vi "Error - Log File.vi"(6 "Clear error?":bool, 8 "error in":errorcluster) -> (0 "error out":errorcluster)   [LabVIEW 2017]
doc: "This SubVI create new or add to existing text file (error_log.txt) data about occured error and current timestamp. Also user can clear occured error by boolean control \"Clear?\"."
uses:
  <vilib>/ErrorRing/Error Ring.xnode
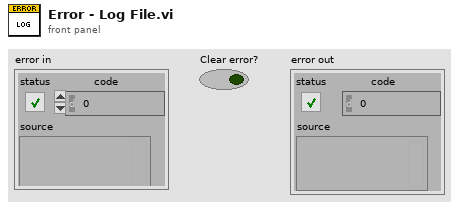
[diagram p1: front panel]
types:
  T1 = enum16{"open", "replace", "create", "open or create", "replace or create", "replace or create with confirmation"}
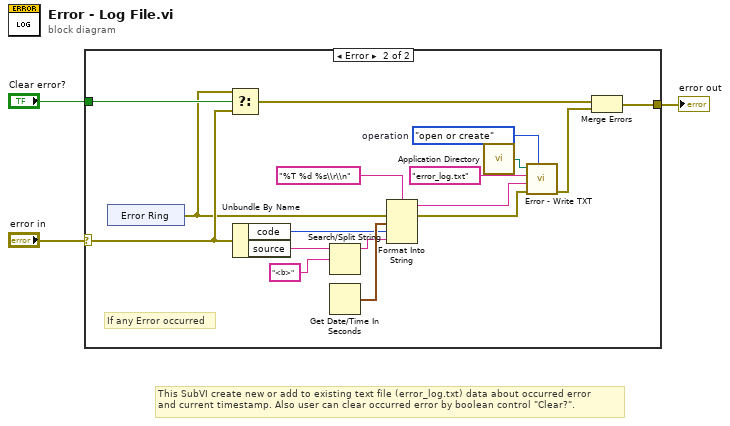
[diagram p0: block diagram]
diagram:
  # "This SubVI create new or add to existing text file (error_log.txt) data about occurred error \nand current timestamp. Also user can clear occurred error by boolean control \"Clear?\"."
  n1 = case shown="Error" "error in" {
    selector: "error in" -> [w4 w13]
    tunnel: [w4 w14] -> w3
    tunnel: "Clear error?" -> [_ w12]
    frame No Error {
      # "If NO Error occurred"
    }
    frame Error {
      w5 = T1."open or create"  # operation
      # "If any Error occurred"
      n2 = xnode "Error Ring"() -> ("error out"=w6:errorcluster)
      n3 = Select(t=w6, s=w12, f=w13) -> (s? t:f=w15:errorcluster)
      n4 = Unbundle By Name(w13) -> ("code"=w19:i32, "source"=w18:string)
      n5 = Search/Split String(string=w18, search string/char (-)="<b>" ("regular expression")) -> (substring before match=w16:string)  [unwired: 1 in, 2 out]
      n6 = Get Date/Time In Seconds() -> (seconds since 1Jan1904=w20:timestamp)
      n7 = Format Into String(format string="%T %d %s\\r\\n", error in=w6, w20, w19, w16) -> (resulting string=w8:string, error out=w10:errorcluster)  [unwired: 1 in]
      n8 = call <vilib>:"Application Directory.vi"() -> ("Application Directory"=w11:path)
      n9 = call "Error - Write TXT.vi"("operation"=w5, "error in"=w10, "text"=w8, "filename.txt"="error_log.txt" ("name or relative path"), "base path"=w11) -> ("error out"=w7:errorcluster)  [unwired: 6 in]
      n10 = Merge Errors(w15, w7) -> (w14:errorcluster)
    }
  }
  "error out" <- w3
